vi "Serialize PAS.vi"() -> ()   [LabVIEW 2012]
uses:
  cPAS.lvclass
  Reusable/PAS/Cell/PAS Cell.lvclass
  Reusable/Switch/Switch.lvclass
  Reusable/PAS/Data/Main/PAS Data.lvclass
  Reusable/PAS/Data/Cell/PAS Cell Data.lvclass
  Data/cPAS Data.lvclass
  Data/cPAS Cell Data/cPAS Cell Data.lvclass
  Reusable/PAS/Main/Controls/period_length.ctl
  Reusable/PAS/Main/Controls/LasLam.ctl
  Reusable/PAS/Main/Controls/Cell Condition.ctl
  Reusable/PAS/Main/Controls/Laser Modulation.ctl
  Reusable/PAS/Cell/FPGA Ctl Params.ctl
  Utilities/FPGA/Controls/FPGAConfig.ctl
  <userlib>/Serialization/Formatter/Formatter.lvclass
  Devices/TE Cooler/TE Cooler.lvclass
  Reusable/Serial IO/Serial IO.lvclass
  Devices/Alicat/Alicat.lvclass
  Devices/Alicat/Controls/Gas.ctl
  Devices/Alicat/Controls/CtlSetup.ctl
  Devices/Alicat/AlicatCommBank/AlicatCommBank.lvclass
panel:
  out "error out":errorcluster
  out "JSON String":string
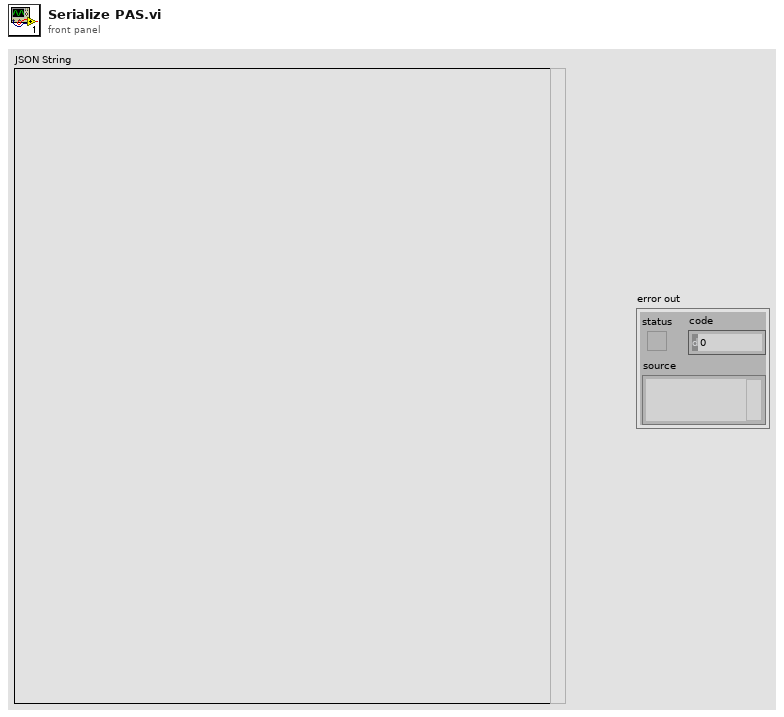
[diagram p1: front panel]
types:
  T1 = typedef "Alicat.lvlib/Alicat.lvclass/CtlSetup.ctl" = cluster{"Name":string, "Address":string, "fullScale":dbl, "Gas":T2}
  T2 = typedef "Alicat.lvlib/Alicat.lvclass/Gas.ctl" = enum16{"Air", "Ar", "CH4", "CO", "CO2", "C2H6", "H2", "He", "N2", "NO", "Ne", "O2", "C3H8", "n-C4H10", "C2H2", "C2H4", "i-C2H10", "Kr", "Xe"}
  T3 = enum16{"No paths embedded", "One path with each object", "All paths with top object"}
  T4 = typedef "FPGAConfig.ctl" = cluster{"Span":cluster{"ch 1":sgl, "ch 2":sgl, "ch 3":sgl, "ch 4":sgl, "ch 5":sgl}, "mod":cluster{"ch 1":T5, "ch 2":T5, "ch 3":T5, "ch 4":T5, "ch 5":T5}}
  T5 = typedef "Laser Modulation.ctl" = enum8{"Sine", "Square"}
  T6 = typedef "Cell Condition.ctl" = enum16{"Dry", "Humidified", "Denuded"}
  T7 = typedef "LasLam.ctl" = enum16{"405", "532", "661"}
  T8 = typedef "period_length.ctl" = cluster{"period":sgl, "length":sgl}
  T9 = cluster{"ch 1":sgl, "ch 2":sgl, "ch 3":sgl, "ch 4":sgl, "ch 5":sgl}
  T10 = cluster{"ch 1":T5, "ch 2":T5, "ch 3":T5, "ch 4":T5, "ch 5":T5}
  T11 = typedef "FPGA Ctl Params.ctl" = cluster{"Mod":T5, "Span":sgl, "f0":sgl}
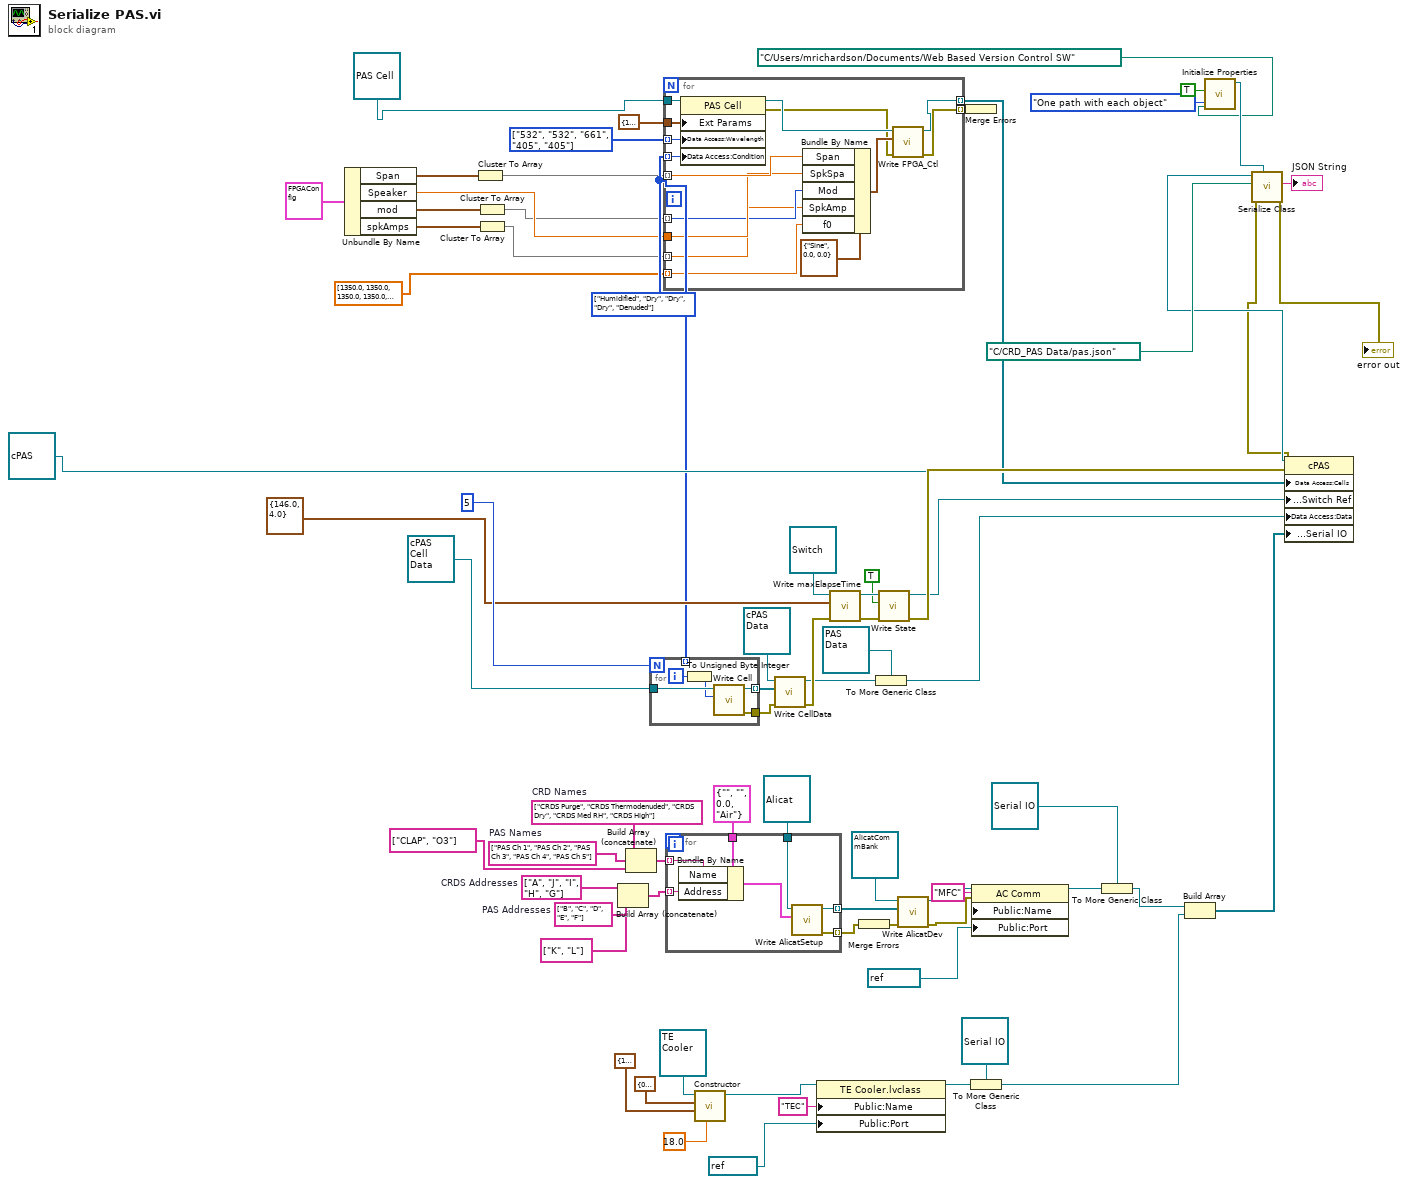
[diagram p0: block diagram]
diagram:
  w21 = string[] ["CRDS Purge", "CRDS Thermodenuded", "CRDS Dry", "CRDS Med RH", "CRDS High"]  # CRD Names
  w23 = string[] ["A", "J", "I", "H", "G"]  # CRDS Addresses
  w19 = string[] ["B", "C", "D", "E", "F"]  # PAS Addresses
  w20 = string[] ["PAS Ch 1", "PAS Ch 2", "PAS Ch 3", "PAS Ch 4", "PAS Ch 5"]  # PAS Names
  w47 = T6[] [enum."Humidified", enum."Dry", enum."Dry", enum."Dry", enum."Denuded"] items=["Dry", "Humidified", "Denuded"]
  w49 = T7[] [enum."532", enum."532", enum."661", enum."405", enum."405"] items=["405", "532", "661"]
  n1 = Unbundle By Name(T4 {"Span"={"ch 1"=3.3, "ch 2"=3.3, "ch 3"=3.0, "ch 4"=3.0, "ch 5"=3.0}, "mod"={"ch 1"=enum."Square", "ch 2"=enum."Square", "ch 3"=enum."Sine", "ch 4"=enum."Square", "ch 5"=enum."Square"}} ("FPGA Output")) -> ("Span"=w46:T9, "Speaker"=w42:sgl, "mod"=w45:T10, "spkAmps"=w44:T9)
  n2 = Cluster To Array(cluster=w46) -> (array=w43:sgl[])
  n3 = Cluster To Array(cluster=w45) -> (array=w41:T5[])
  n4 = Cluster To Array(cluster=w44) -> (array=w40:sgl[])
  n5 = Build Array (concatenate)(w23, w19, string[] ["K", "L"] ("array")) -> (w12:string[])
  n6 = Build Array (concatenate)(w21, w20, string[] ["CLAP", "O3"] ("array")) -> (w22:string[])
  n7 = for {
    N: 5 ("default value") -> [_]
    tunnel: refnum<class "cPAS Cell Data.lvclass"> refnum ("cPAS Cell") -> [w78]
    tunnel: [w77] -> w66 mode=indexing
    tunnel: [w74] -> w65
    tunnel: w47 -> [_] mode=indexing
    i -> [w76]
    n8 = To Unsigned Byte Integer(number=w76) -> (unsigned 8bit integer=w75:u8)
    n9 = call "Write Cell.vi"("Cell"=w75, "PAS Cell Data in"=w78) -> ("error out"=w74:errorcluster, "PAS Cell Data out"=w77:refnum<class "cPAS Cell Data.lvclass">)  [unwired: 8 in]
  }
  n10 = for {
    tunnel: [w85] -> w51 mode=indexing
    tunnel: refnum<class "PAS Cell.lvclass"> refnum ("Base PAS.lvlib:PAS Cell") -> [w93]
    tunnel: cluster{"slope":sgl, "zero":sgl} {"slope"=1.0, "zero"=0.0} ("Ext Params") -> [w92]
    tunnel: w49 -> [w91] mode=indexing
    tunnel: w47 -> [w90] mode=indexing
    tunnel: [w79] -> w37 mode=indexing
    tunnel: w43 -> [w84] mode=indexing
    tunnel: w42 -> [w83]
    tunnel: w41 -> [w82] mode=indexing
    tunnel: w40 -> [w81] mode=indexing
    tunnel: dbl[] [1350.0, 1350.0, 1350.0, 1350.0, 1350.0] -> [w80] mode=indexing
    n11 = property class="PAS Cell"(reference=w93, "Ext Params"=w92, "Data Access:Wavelength"=w91, "Data Access:Condition"=w90) -> (reference out=w87:refnum<class "PAS Cell.lvclass">, error out=w86:errorcluster)  [unwired: 1 in]
    n12 = Bundle By Name(cluster=T11 {"Mod"=enum."Sine", "Span"=0.0, "f0"=0.0} ("FPGA_Ctl"), "Span"=w84, "SpkSpa"=w83, "Mod"=w82, "SpkAmp"=w81, "f0"=w80) -> (w89:T11)
    n13 = call "Write FPGA_Ctl.vi"("error in (no error)"=w86, "FPGA_Ctl"=w89, "PAS Cell in"=w87) -> ("error out"=w85:errorcluster, "PAS Cell out"=w79:refnum<class "PAS Cell.lvclass">)  [unwired: 7 in]
  }
  n14 = for {
    tunnel: T1 {"Name"="", "Address"="", "fullScale"=0.0, "Gas"=enum."Air"} ("AlicatSetup") -> [w98]
    tunnel: w22 -> [w97] mode=indexing
    tunnel: refnum<class "Alicat.lvclass"> refnum ("Alicat") -> [w100]
    tunnel: [w99] -> w15 mode=indexing
    tunnel: w12 -> [w96] mode=indexing
    tunnel: [w94] -> w17 mode=indexing
    n15 = Bundle By Name(cluster=w98, "Name"=w97, "Address"=w96) -> (w95:T1)
    n16 = call "Write AlicatSetup.vi"("AlicatSetup"=w95, "Alicat in"=w100) -> ("error out"=w94:errorcluster, "Alicat out"=w99:refnum<class "Alicat.lvclass">)  [unwired: 8 in]
  }
  n17 = call "Constructor.vi"("TSP"=sgl 18.0, "PID Params"=cluster{"P":sgl, "I":sgl, "D":sgl} {"P"=1.0, "I"=0.75, "D"=0.0}, "Ctl Params"=cluster{"htx":sgl, "clx":sgl} {"htx"=0.0, "clx"=1.0}, "TE Cooler in"=refnum<class "TE Cooler.lvclass"> refnum ("TE Cooler.lvlib:TE Cooler.lvclass")) -> ("TE Cooler out"=w27:refnum<class "TE Cooler.lvclass">)  [unwired: 6 in, 1 out]
  n18 = call "Write CellData.vi"("error in"=w65, "CellData"=w66, "PAS Data in"=refnum<class "cPAS Data.lvclass"> refnum ("cPAS Data")) -> ("error out"=w63:errorcluster, "PAS Data out"=w60:refnum<class "cPAS Data.lvclass">)  [unwired: 7 in]
  n19 = property class="TE Cooler.lvclass"(reference=w27, "Public:Name"="TEC" ("Name"), "Public:Port"=refnum<visa-resource-name> "TEC" ("Port")) -> (reference out=w24:refnum<class "TE Cooler.lvclass">)  [unwired: 1 in, 1 out]
  n20 = call "Write maxElapseTime.vi"("error in"=w63, "maxElapsedTime"=T8 {"period"=146.0, "length"=4.0} ("f0Check"), "Switch in"=refnum<class "Switch.lvclass"> refnum ("Switch.lvclass")) -> ("error out"=w67:errorcluster, "Switch out"=w69:refnum<class "Switch.lvclass">)  [unwired: 7 in]
  n21 = Merge Errors(w17) -> (w18:errorcluster)
  n22 = To More Generic Class(target class=refnum<class "PAS Data.lvclass"> refnum ("Data"), reference=w60) -> (generic class reference=w52:refnum<class "PAS Data.lvclass">)
  n23 = call-dynamic "Write State.vi"("error in"=w67, "State"=TRUE, "Switch in"=w69) -> ("error out"=w62:errorcluster, "Switch out"=w59:refnum<class "Switch.lvclass">)  [unwired: 7 in]
  n24 = call "Write AlicatDev.vi"("error in"=w18, "AlicatDev"=w15, "AlicatCommBank in"=refnum<class "AlicatCommBank.lvclass"> refnum) -> ("error out"=w6:errorcluster, "AlicatCommBank out"=w9:refnum<class "AlicatCommBank.lvclass">)  [unwired: 7 in]
  n25 = Merge Errors(w51) -> ()  [unwired: 1 out]
  n26 = To More Generic Class(target class=refnum<class "Serial IO.lvclass"> refnum ("Serial IO.lvclass"), reference=w24) -> (generic class reference=w2:refnum<class "Serial IO.lvclass">)
  n27 = property class="AC Comm"(reference=w9, error in=w6, "Public:Name"="MFC" ("Name"), "Public:Port"=refnum<visa-resource-name> "MFC" ("Port")) -> (reference out=w4:refnum<class "AlicatCommBank.lvclass">)  [unwired: 1 out]
  n28 = To More Generic Class(target class=refnum<class "Serial IO.lvclass"> refnum ("Serial IO.lvclass"), reference=w4) -> (generic class reference=w3:refnum<class "Serial IO.lvclass">)
  n29 = Build Array(w3, w2) -> (w1:refnum<class "Serial IO.lvclass">[])
  n30 = call <userlib>:"Initialize Properties.vi"("Absolute Path For Dynamic Loading"=path "C:/Users/mrichardson/Documents/Web Based Version Control SW", "Path Embedding"=T3."One path with each object", "Include all fields?"=TRUE) -> ("Formatter out"=w36:refnum<class "Formatter.lvclass">)  [unwired: 8 in]
  n31 = property class="cPAS"(reference=refnum<class "cPAS.lvclass"> refnum ("cPAS"), error in=w62, "Data Access:Cells"=w37, "Data Access:Switch Ref"=w59, "Data Access:Data"=w52, "Data Access:Serial IO"=w1) -> (reference out=w54:refnum<class "cPAS.lvclass">, error out=w53:errorcluster)
  n32 = call-dynamic "Serialize Class.vi"("Formatter"=w36, "error in"=w53, "file path"=path "C:/CRD_PAS Data/pas.json", "Instrument in"=w54) -> ("error out"=→"error out":errorcluster, "JSON String"=→"JSON String":string)  [unwired: 5 in, 1 out]
